vi "Find Shift.vi"(11 "Shift Info":string[][](array[string])) -> (2 "Shift Time":string, 3 "Shift Name":string)   [LabVIEW 2017]
panel:
  out "Start Time":string="10:00:00 AM"
  out "End Time":string="5:00:00 PM"
  out "In Range?":bool
  out "output 3":timestamp
  out "output 2":timestamp
  out "resulting string":string
  out "output 1":timestamp
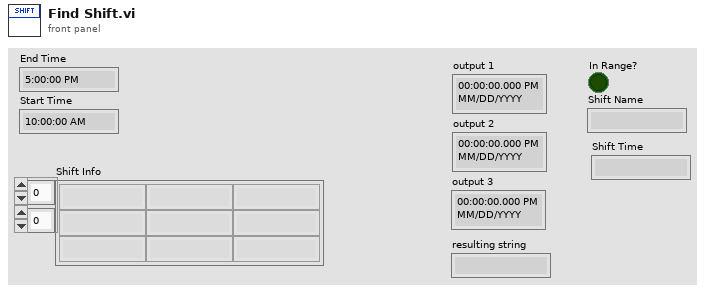
[diagram p1: front panel]
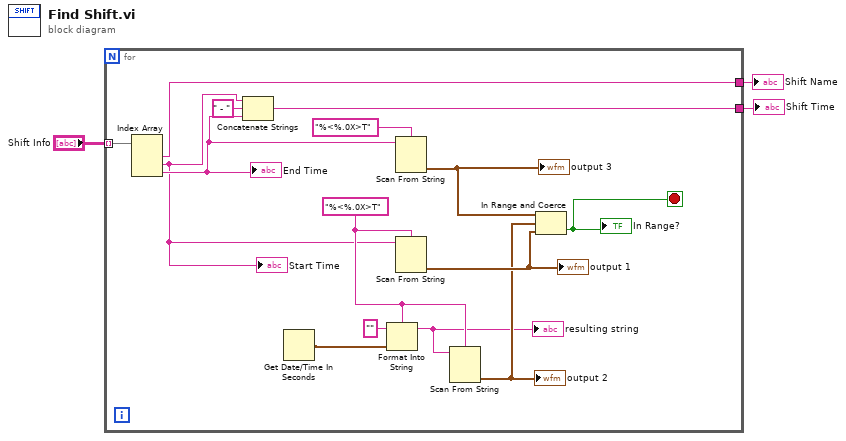
[diagram p0: block diagram]
diagram:
  n1 = for {
    tunnel: "Shift Info" -> [w13] mode=indexing
    tunnel: [w11] -> w2
    tunnel: [w8] -> w1
    stop <- w12 stop-if-true
    w6 = "%<%.0X>T" ("format string")
    n2 = Index Array(array=w13) -> (element #1=w11:string, element #2=w4:string, element #3=w10:string)  [unwired: 3 in]
    "End Time" <- w10
    "Start Time" <- w4
    n3 = Concatenate Strings(w4, " - " ("string"), w10) -> (w8:string)
    n4 = Get Date/Time In Seconds() -> (seconds since 1Jan1904=w14:timestamp)
    n5 = Format Into String(format string=w6, initial string="", w14) -> (resulting string=w5:string)  [unwired: 1 in, 1 out]
    "resulting string" <- w5
    n6 = Scan From String(format string="%<%.0X>T", input string=w10) -> (output 1=w17:timestamp)  [unwired: 3 in, 3 out]
    "output 3" <- w17
    n7 = Scan From String(format string=w6, input string=w4) -> (output 1=w16:timestamp)  [unwired: 3 in, 3 out]
    "output 1" <- w16
    n8 = Scan From String(format string=w6, input string=w5) -> (output 1=w15:timestamp)  [unwired: 3 in, 3 out]
    "output 2" <- w15
    n9 = In Range and Coerce(upper limit=w17, x=w15, lower limit=w16) -> (In Range?=w12:bool)  [unwired: 1 out]
    "In Range?" <- w12
  }
  "Shift Name" <- w2
  "Shift Time" <- w1
